vi "Begin.vi"(8 "error in":errorcluster) -> (0 "error out":errorcluster)   [LabVIEW 2016]
doc: "Called before other user functions, this VI is expected to open initial I/O refnums, load in file data, and do all program initialization. Notice that the <B>error out</B> terminal is simply used for data flow. Wiring it to other structures or subVIs ensures that this VI runs first."
uses:
  <vilib>/Rock Robotics/WPI/DriverStation/WPI_DriverStationRobotMode2.ctl
  <vilib>/Rock Robotics/WPI/Joystick/WPI_JoystickDeviceEnum.ctl
  <vilib>/Rock Robotics/SystemInterfaces/AI/FPGA_AIChannel.ctl
  <vilib>/Rock Robotics/SystemInterfaces/DIO/FPGA_DIOPWMChannel.ctl
  <vilib>/Rock Robotics/WPI/ThirdParty/CanMotor/TalonSRX/WPI_CANTalonSRX_APIControlMode.ctl
  <vilib>/Rock Robotics/WPI/ThirdParty/CanMotor/TalonSRX/WPI_CANTalonSRX_BrakeOverride.ctl
  <vilib>/Rock Robotics/SystemInterfaces/AI/FPGA_AIGyroChannel.ctl
  <vilib>/Rock Robotics/Network Tables/NT Write String Array.vi
  Robot Global Data.vi
  <vilib>/Rock Robotics/WPI/MotorControl/WPI_MotorControlOpen SPARK.vi
  <vilib>/Rock Robotics/Network Tables/NT Write Boolean.vi
  <vilib>/Rock Robotics/WPI/Ultrasonic/WPI_SonarMB1010AnalogOpen.vi
  <vilib>/Rock Robotics/WPI/Ultrasonic/WPI_SonarMB1010AnalogRefNum Registry Set.vi
  <vilib>/Rock Robotics/WPI/Switch/WPI_SwitchOpenLimit.vi
  <vilib>/Rock Robotics/SystemInterfaces/DIO/FPGA_DIOChannel.ctl
  2039lib.lvlib
panel:
  in  "Robot Mode":T1
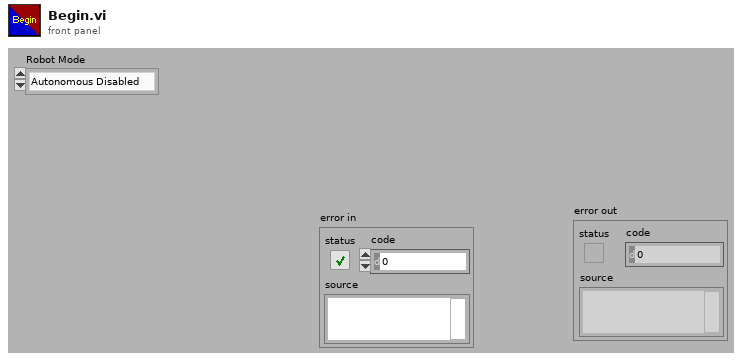
[diagram p1: front panel]
types:
  T1 = typedef "WPI_DriverStationRobotMode2.ctl" = enum16{"Autonomous Disabled", "Autonomous Enabled", "Teleop Disabled", "Teleop Enabled", "Disconnected", "Finish", "Test Disabled", "Test Enabled", "Emergency Stopped"}
  T2 = typedef "FPGA_DIOPWMChannel.ctl" = enum8{"PWM 0", "PWM 1", "PWM 2", "PWM 3", "PWM 4", "PWM 5", "PWM 6", "PWM 7", "PWM 8", "PWM 9", "PWM MXP 0", "PWM MXP 1", "PWM MXP 2", "PWM MXP 3", "PWM MXP 4", "PWM MXP 5", "PWM MXP 6", "PWM MXP 7", "PWM MXP 8", "PWM MXP 9", "Invalid"}
  T3 = enum16{"Driver Control", "Gear Coarse Adjust", "Gear Fine Adjust"}
  T4 = typedef "FPGA_AIGyroChannel.ctl" = enum8{"AI 0", "AI 1", "Invalid"}
  T5 = typedef "WPI_CANTalonSRX_BrakeOverride.ctl" = enum8{"No Override", "Override to Coast", "Override to Brake"}
  T6 = typedef "WPI_CANTalonSRX_APIControlMode.ctl" = enum8{"Percent VBus", "Speed", "Position", "Slave", "Unchanged / Invalid", "Voltage Compensation", "Current", "Motion Profile", "Motion Magic"}
  T7 = typedef "WPI_JoystickDeviceEnum.ctl" = enum16{"USB 0", "USB 1", "USB 2", "USB 3", "USB 4", "USB 5"}
  T8 = typedef "FPGA_AIChannel.ctl" = enum8{"AI 0", "AI 1", "AI 2", "AI 3", "AI MXP 0", "AI MXP 1", "AI MXP 2", "AI MXP 3", "Invalid"}
  T9 = typedef "WPI_MotorControlDeviceRef.ctl" = cluster{"DeviceStatus":errorcluster, "Type":T10, "PWM":cluster{"PWM Channel":T2, "DeadBand":T11}, "CAN":cluster{"Device Number":u8, "SetOutput VI Ref":variant, "GetOutput VI Ref":variant, "Enable VI Ref":variant, "Disable VI Ref":variant, "Data":variant}, "Invert":bool}
  T10 = typedef "WPI_MotorControlType.ctl" = enum16{"PWM", "CAN"}
  T11 = typedef "WPI_PWMDeadband.ctl" = cluster{"Name":string, "maxPositivePwm":i32, "minPositivePwm":i32, "centerPwm":i32, "maxNegativePwm":i32, "minNegativePwm":i32, "angularRange":u16}
  T12 = typedef "FPGA_DIOChannel.ctl" = enum8{"DIO 0", "DIO 1", "DIO 2", "DIO 3", "DIO 4", "DIO 5", "DIO 6", "DIO 7", "DIO 8", "DIO 9", "DIO MXP 0", "DIO MXP 1", "DIO MXP 2", "DIO MXP 3", "DIO MXP 4", "DIO MXP 5", "DIO MXP 6", "DIO MXP 7", "DIO MXP 8", "DIO MXP 9", "DIO MXP 10", "DIO MXP 11", "DIO MXP 12", "DIO MXP 13", "DIO MXP 14", "DIO MXP 15", "SPI Port CS1", "SPI Port CS2", "SPI Port CS3", "SPI Port MISO", "SPI Port MOSI", "Invalid"}
  T13 = typedef "WPI_DigitalInputDevRef.ctl" = cluster{"DevStatus":errorcluster, "DIO Channel":T12}
  T14 = typedef "WPI_SwitchDevRef.ctl" = cluster{"DevStatus":errorcluster, "DIO Channel":T12, "CntIndex":T15, "Normally Closed":bool}
  T15 = typedef "FPGA_CounterCtrSystemIndex.ctl" = enum8{"Ctr 0", "Ctr 1", "Ctr 2", "Ctr 3", "Ctr 4", "Ctr 5", "Ctr 6", "Ctr 7", "Invalid"}
  T16 = typedef "WPI_JoystickDevRef.ctl" = cluster{"Device":T7}
  T17 = typedef "WPI_SonarMB1010AnalogDeviceRef.ctl" = cluster{"AIDeviceRef":T18, "Scaling factor (V/in)":dbl, "Average Bits":u8}
  T18 = typedef "WPI_AnalogChannelDevRef.ctl" = cluster{"DevStatus":errorcluster, "Analog Channel":T8}
  T19 = typedef "WPI_ServoDeviceRef.ctl" = cluster{"DeviceStatus":errorcluster, "PWM Channel":T2, "DeadBand":T11}
  T20 = typedef "WPI_GyroDevRef.ctl" = cluster{"DevStatus":errorcluster, "Analog Channel":T8, "Offset":dbl, "Gain (VoltsPerDegree/Second)":dbl, "Gyro Type":enum16{"Analog", "XRS450"}, "Handle":i32, "SPI Bus":T21, "Device Found":bool, "Sample Rate":dbl, "Calibrate On Open":bool}
  T21 = typedef "spi_bus.ctl" = enum16{"SPI On-Board, CS0", "SPI On-Board, CS1", "SPI On-Board, CS2", "SPI On-Board, CS3", "SPI MXP", "Invalid"}
  T22 = typedef "WPI_AccelerometerDevRef.ctl" = cluster{"DevStatus":errorcluster, "Scaling":T23, "Analog Channels":T24, "I2C Bus":T25, "SPI Bus":T21, "Accel Range":T26, "ADXL Axes":T27, "Handle":i32, "Device Address":u8, "Accel Type":enum16{"Analog", "ADXL345 I2C", "ADXL345 SPI", "Internal", "ADXL362 SPI"}}
  T23 = typedef "WPI_AccelerometerScaling.ctl" = cluster{"Gain (VoltsPerG)":dbl, "Center Voltage":dbl}
  T24 = typedef "WPI_AccelerometerAnalogChannels.ctl" = cluster{"X-Axis":T8, "Y-Axis":T8, "Z-Axis":T8}
  T25 = typedef "i2c_bus.ctl" = enum16{"I2C On-Board", "I2C MXP", "Invalid"}
  T26 = typedef "ADXL345 Range.ctl" = u8
  T27 = typedef "WPI_AccelerometerADXL345 Axes.ctl" = cluster{"X-Axis":bool, "Y-Axis":bool, "Z-Axis":bool}
  T28 = cluster{"GyroDevRef":T20, "AccelerometerDevRef":T22}
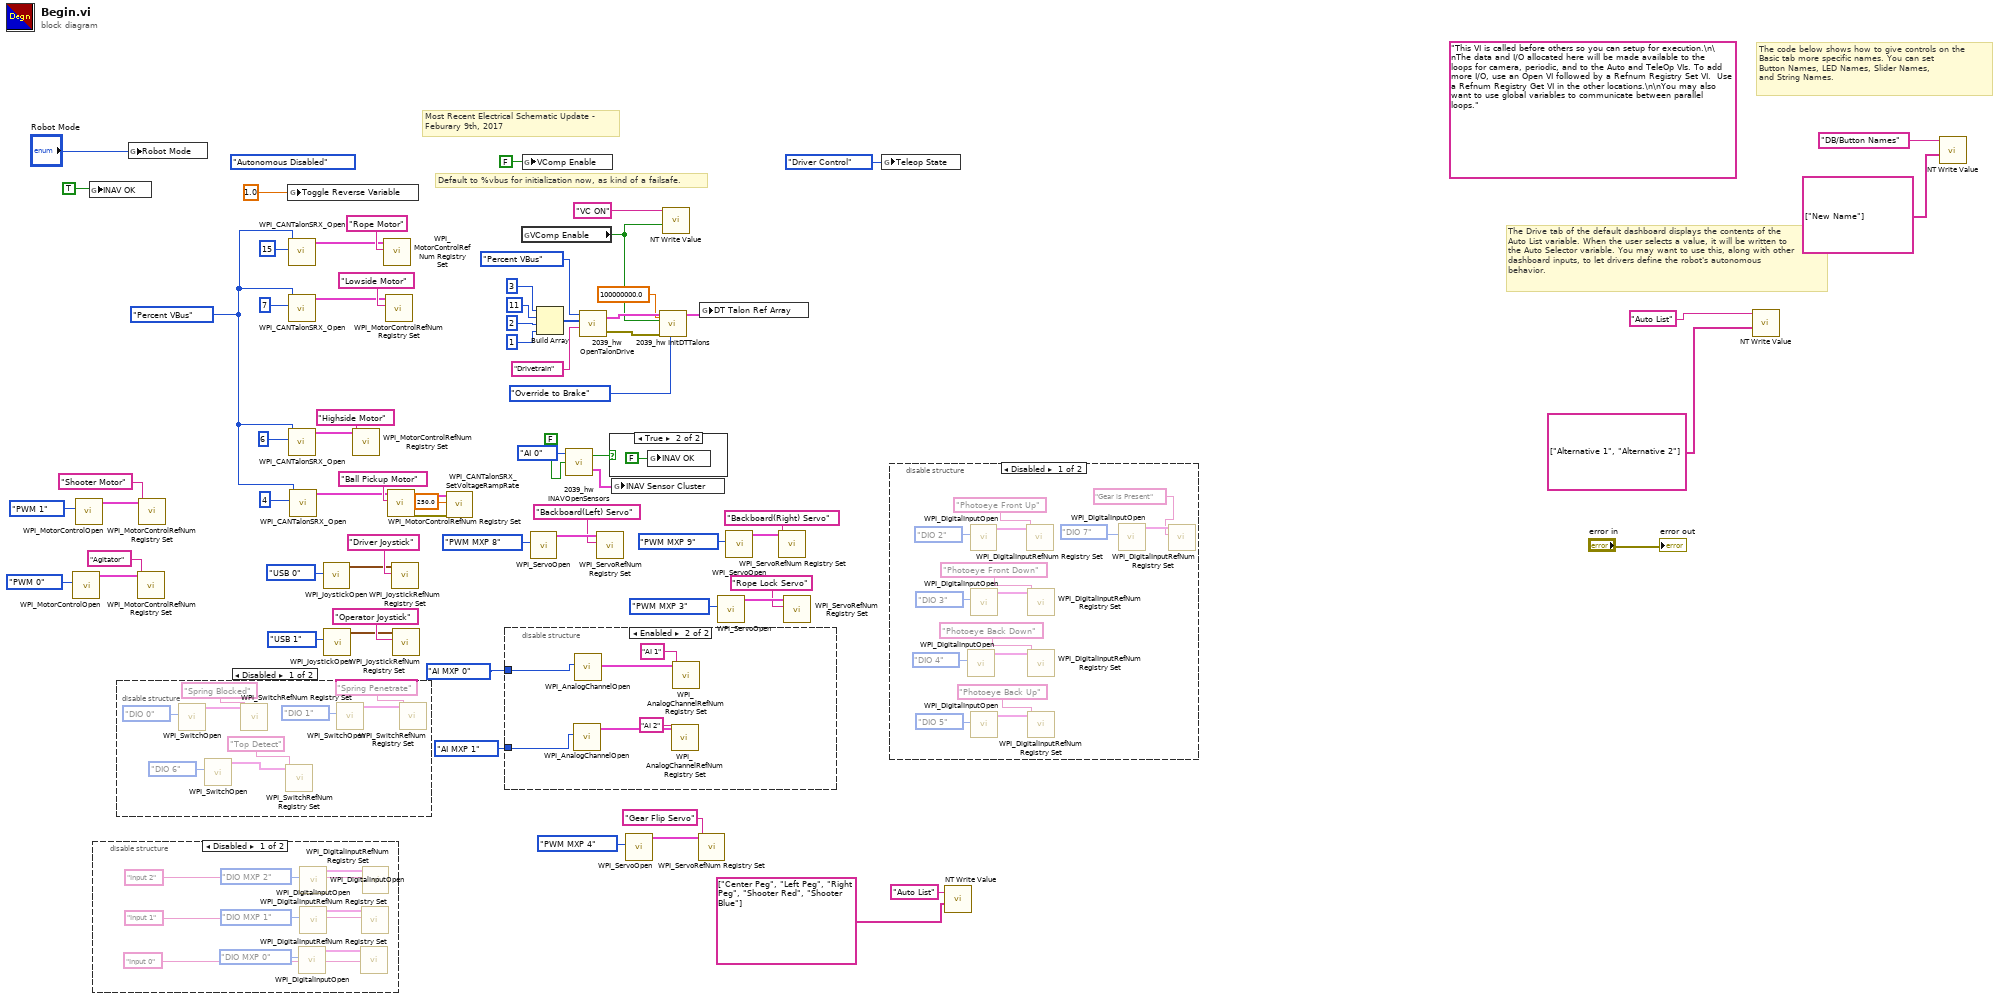
[diagram p0: block diagram]
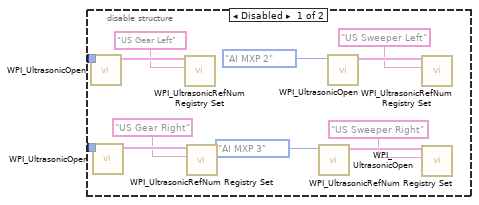
[diagram p4: hidden frame]
diagram:
  w50 = WPI_CANTalonSRX_APIControlMode."Percent VBus" ("Control Mode")
  (unwired) WPI_DriverStationRobotMode2."Autonomous Disabled" ("Robot Mode")
  (unwired) "This VI is called before others so you can setup for execution.\n\nThe data and I/O allocated here will be made available to the loops for camera, periodic, and to the Auto and TeleOp VIs. To add more I/O, use an Open VI followed by a Refnum Registry Set VI.  Use a Refnum Registry Get VI in the other locations.\n\nYou may also want to use global variables to communicate between parallel loops."
  # "Default to %vbus for initialization now, as kind of a failsafe."
  # "Most Recent Electrical Schematic Update -\nFeburary 9th, 2017"
  # "The Drive tab of the default dashboard displays the contents of the\nAuto List variable. When the user selects a value, it will be written to\nthe Auto Selector variable. You may want to use this, along with other\ndashboard inputs, to let drivers define the robot's autonomous\nbehavior."
  # "The code below shows how to give controls on the\nBasic tab more specific names. You can set\nButton Names, LED Names, Slider Names,\nand String Names."
  n1 = call-poly <vilib>:"WPI_MotorControlOpen.vi"("PWM Channel"=FPGA_DIOPWMChannel."PWM 0") -> ("MotorControlDeviceRef"=w6:T9)  [unwired: 9 in, 1 out]
  n2 = call-poly <vilib>:"WPI_MotorControlOpen.vi"("PWM Channel"=FPGA_DIOPWMChannel."PWM 1") -> ("MotorControlDeviceRef"=w7:T9)  [unwired: 9 in, 1 out]
  n3 = global write "Robot Global Data.vi" "INAV OK"(TRUE) -> ()
  n4 = disable-structure shown="Disabled" {
    frame Disabled {
      n5 = call <vilib>:"WPI_DigitalInputOpen.vi"("DIO Channel"=FPGA_DIOChannel."DIO MXP 0") -> ("DigitalInputDevRef"=w77:T13)  [unwired: 9 in, 1 out]
      n6 = call <vilib>:"WPI_DigitalInputOpen.vi"("DIO Channel"=FPGA_DIOChannel."DIO MXP 2") -> ("DigitalInputDevRef"=w76:T13)  [unwired: 9 in, 1 out]
      n7 = call <vilib>:"WPI_DigitalInputOpen.vi"("DIO Channel"=FPGA_DIOChannel."DIO MXP 1") -> ("DigitalInputDevRef"=w78:T13)  [unwired: 9 in, 1 out]
      n8 = call <vilib>:"WPI_DigitalInputRefNum Registry Set.vi"("refnum name"="Input 0", "DigitalInputDevRef"=w77) -> ()  [unwired: 8 in, 2 out]
      n9 = call <vilib>:"WPI_DigitalInputRefNum Registry Set.vi"("refnum name"="Input 1", "DigitalInputDevRef"=w78) -> ()  [unwired: 8 in, 2 out]
      n10 = call <vilib>:"WPI_DigitalInputRefNum Registry Set.vi"("refnum name"="Input 2", "DigitalInputDevRef"=w76) -> ()  [unwired: 8 in, 2 out]
    }
    frame Enabled {
    }
  }
  n11 = disable-structure shown="Disabled" {
    frame Disabled {
      n12 = call-poly <vilib>:"WPI_SwitchOpen.vi"("DIO Channel"=FPGA_DIOChannel."DIO 0") -> ("SwitchDevRef"=w90:T14)  [unwired: 9 in, 1 out]
      n13 = call-poly <vilib>:"WPI_SwitchOpen.vi"("DIO Channel"=FPGA_DIOChannel."DIO 6") -> ("SwitchDevRef"=w84:T14)  [unwired: 9 in, 1 out]
      n14 = call <vilib>:"WPI_SwitchRefNum Registry Set.vi"("refnum name"="Spring Blocked", "SwitchDevRef"=w90) -> ()  [unwired: 8 in, 2 out]
      n15 = call <vilib>:"WPI_SwitchRefNum Registry Set.vi"("refnum name"="Top Detect", "SwitchDevRef"=w84) -> ()  [unwired: 8 in, 2 out]
      n16 = call-poly <vilib>:"WPI_SwitchOpen.vi"("DIO Channel"=FPGA_DIOChannel."DIO 1") -> ("SwitchDevRef"=w87:T14)  [unwired: 9 in, 1 out]
      n17 = call <vilib>:"WPI_SwitchRefNum Registry Set.vi"("refnum name"="Spring Penetrate", "SwitchDevRef"=w87) -> ()  [unwired: 8 in, 2 out]
    }
    frame Enabled {
    }
  }
  n18 = global write "Robot Global Data.vi" "Robot Mode"("Robot Mode") -> ()
  n19 = call <vilib>:"WPI_MotorControlRefNum Registry Set.vi"("refnum name"="Agitator", "MotorControlDevRef"=w6) -> ()  [unwired: 8 in, 2 out]
  n20 = call <vilib>:"WPI_MotorControlRefNum Registry Set.vi"("refnum name"="Shooter Motor", "MotorControlDevRef"=w7) -> ()  [unwired: 8 in, 2 out]
  n21 = global write "Robot Global Data.vi" "Toggle Reverse Variable"(1.0 ("Toggle Reverse Variable")) -> ()
  n22 = call <vilib>:"WPI_CANTalonSRX_Open.vi"("Device Number"=15, "Control Mode"=w50) -> ("CAN Talon SRX Ref"=w44:T9)  [unwired: 8 in, 1 out]
  n23 = call <vilib>:"WPI_CANTalonSRX_Open.vi"("Device Number"=7, "Control Mode"=w50) -> ("CAN Talon SRX Ref"=w43:T9)  [unwired: 8 in, 1 out]
  n24 = call <vilib>:"WPI_CANTalonSRX_Open.vi"("Device Number"=6, "Control Mode"=w50) -> ("CAN Talon SRX Ref"=w42:T9)  [unwired: 8 in, 1 out]
  n25 = call <vilib>:"WPI_CANTalonSRX_Open.vi"("Device Number"=4, "Control Mode"=w50) -> ("CAN Talon SRX Ref"=w41:T9)  [unwired: 8 in, 1 out]
  n26 = call <vilib>:"WPI_JoystickOpen.vi"("JoystickDevice"=WPI_JoystickDeviceEnum."USB 0") -> ("JoystickDevRef"=w71:T16)  [unwired: 10 in]
  n27 = call <vilib>:"WPI_JoystickOpen.vi"("JoystickDevice"=WPI_JoystickDeviceEnum."USB 1") -> ("JoystickDevRef"=w61:T16)  [unwired: 10 in]
  n28 = call <vilib>:"WPI_MotorControlRefNum Registry Set.vi"("refnum name"="Highside Motor", "MotorControlDevRef"=w42) -> ()  [unwired: 8 in, 2 out]
  n29 = call <vilib>:"WPI_MotorControlRefNum Registry Set.vi"("refnum name"="Rope Motor", "MotorControlDevRef"=w44) -> ()  [unwired: 8 in, 2 out]
  n30 = call <vilib>:"WPI_MotorControlRefNum Registry Set.vi"("refnum name"="Lowside Motor", "MotorControlDevRef"=w43) -> ()  [unwired: 8 in, 2 out]
  n31 = call <vilib>:"WPI_MotorControlRefNum Registry Set.vi"("refnum name"="Ball Pickup Motor", "MotorControlDevRef"=w41) -> ("error out"=w11:errorcluster, "MotorControlDevRef"=w12:T9)  [unwired: 8 in]
  n32 = call <vilib>:"WPI_JoystickRefNum Registry Set.vi"("refnum name"="Driver Joystick", "JoystickDevRef"=w71) -> ()  [unwired: 8 in, 2 out]
  n33 = call <vilib>:"WPI_JoystickRefNum Registry Set.vi"("refnum name"="Operator Joystick", "JoystickDevRef"=w61) -> ()  [unwired: 8 in, 2 out]
  n34 = call <vilib>:"WPI_CANTalonSRX_SetVoltageRampRate.vi"("error in (no error)"=w11, "Throttle Ramp Rate (percent/s)"=250.0, "CAN Talon SRX Ref"=w12) -> ()  [unwired: 7 in, 2 out]
  n35 = disable-structure shown="Enabled" {
    disable-tunnel: FPGA_AIChannel."AI MXP 0" ("Analog Channel") -> [w102 w107]
    disable-tunnel: FPGA_AIChannel."AI MXP 1" ("Analog Channel") -> [w99 w108]
    frame Disabled {
      n36 = call-poly <vilib>:"WPI_UltrasonicOpen.vi"("Analog Channel"=w102) -> ("SonarMB1010AnalogDevRef"=w101:T17)  [unwired: 9 in, 1 out]
      n37 = call-poly <vilib>:"WPI_UltrasonicOpen.vi"("Analog Channel"=w99) -> ("SonarMB1010AnalogDevRef"=w98:T17)  [unwired: 9 in, 1 out]
      n38 = call-poly <vilib>:"WPI_UltrasonicRefNum Registry Set.vi"("refnum name"="US Gear Left", "SonarMB1010AnalogDevRef"=w101) -> ()  [unwired: 8 in, 2 out]
      n39 = call-poly <vilib>:"WPI_UltrasonicRefNum Registry Set.vi"("refnum name"="US Gear Right", "SonarMB1010AnalogDevRef"=w98) -> ()  [unwired: 8 in, 2 out]
      n40 = call-poly <vilib>:"WPI_UltrasonicOpen.vi"("Analog Channel"=FPGA_AIChannel."AI MXP 3") -> ("SonarMB1010AnalogDevRef"=w92:T17)  [unwired: 9 in, 1 out]
      n41 = call-poly <vilib>:"WPI_UltrasonicOpen.vi"("Analog Channel"=FPGA_AIChannel."AI MXP 2") -> ("SonarMB1010AnalogDevRef"=w95:T17)  [unwired: 9 in, 1 out]
      n42 = call-poly <vilib>:"WPI_UltrasonicRefNum Registry Set.vi"("refnum name"="US Sweeper Left", "SonarMB1010AnalogDevRef"=w95) -> ()  [unwired: 8 in, 2 out]
      n43 = call-poly <vilib>:"WPI_UltrasonicRefNum Registry Set.vi"("refnum name"="US Sweeper Right", "SonarMB1010AnalogDevRef"=w92) -> ()  [unwired: 8 in, 2 out]
    }
    frame Enabled {
      n44 = call <vilib>:"WPI_AnalogChannelOpen.vi"("Analog Channel"=w108) -> ("AIDeviceRef"=w106:T18)  [unwired: 9 in, 1 out]
      n45 = call <vilib>:"WPI_AnalogChannelOpen.vi"("Analog Channel"=w107) -> ("AIDeviceRef"=w105:T18)  [unwired: 9 in, 1 out]
      n46 = call <vilib>:"WPI_AnalogChannelRefNum Registry Set.vi"("refnum name"="AI 2", "AIDeviceRef"=w106) -> ()  [unwired: 8 in, 2 out]
      n47 = call <vilib>:"WPI_AnalogChannelRefNum Registry Set.vi"("refnum name"="AI 1", "AIDeviceRef"=w105) -> ()  [unwired: 8 in, 2 out]
    }
  }
  n48 = global read "Robot Global Data.vi" "VComp Enable"() -> (w17:bool)
  n49 = global write "Robot Global Data.vi" "VComp Enable"(FALSE) -> ()
  n50 = call <vilib>:"WPI_ServoOpen.vi"("PWM Channel"=FPGA_DIOPWMChannel."PWM MXP 8") -> ("ServoDeviceRef"=w20:T19)  [unwired: 9 in, 1 out]
  n51 = Build Array(u8 3 ("Device Number"), u8 11 ("Device Number"), u8 2 ("Device Number"), u8 1 ("Device Number")) -> (w34:u8[])
  n52 = call "2039_hw INAVOpenSensors.vi"("Use External Accel"=FALSE, "Gyroscope Analog Channel"=FPGA_AIGyroChannel."AI 0") -> ("INAV Sensor Cluster"=w1:T28, "INAV Not OK"=w24:bool)  [unwired: 1 in]
  n53 = call "2039_hw OpenTalonDrive.vi"("refnum name"="Drivetrain", "CAN IDs"=w34, "Control Mode"=WPI_CANTalonSRX_APIControlMode."Percent VBus") -> ("error out"=w30:errorcluster, "Drivetrain Talon SRX Ref Array"=w31:T9[])  [unwired: 1 in]
  n54 = call <vilib>:"WPI_ServoRefNum Registry Set.vi"("refnum name"="Backboard(Left) Servo", "ServoDeviceRef"=w20) -> ()  [unwired: 8 in, 2 out]
  n55 = case shown="True" w24 {
    frame False {
    }
    frame True {
      n56 = global write "Robot Global Data.vi" "INAV OK"(FALSE) -> ()
    }
  }
  n57 = global write "Robot Global Data.vi" "INAV Sensor Cluster"(w1) -> ()
  n58 = call <vilib>:"WPI_ServoOpen.vi"("PWM Channel"=FPGA_DIOPWMChannel."PWM MXP 4") -> ("ServoDeviceRef"=w14:T19)  [unwired: 9 in, 1 out]
  n59 = call "2039_hw InitDTTalons.vi"("Brake / Coast Mode"=WPI_CANTalonSRX_BrakeOverride."Override to Brake", "Ramp Rate (Percent/s)"=100000000.0, "error in (no error)"=w30, "Enable VComp"=w17, "DT Talon Ref Array"=w31) -> ("DT Talon Ref Array"=w22:T9[])  [unwired: 5 in, 1 out]
  n60 = call-poly <vilib>:"NT Write Value.vi"("Boolean"=w17, "Name"="VC ON") -> ()  [unwired: 9 in, 1 out]
  n61 = call <vilib>:"WPI_ServoRefNum Registry Set.vi"("refnum name"="Gear Flip Servo", "ServoDeviceRef"=w14) -> ()  [unwired: 8 in, 2 out]
  n62 = global write "Robot Global Data.vi" "DT Talon Ref Array"(w22) -> ()
  n63 = call <vilib>:"WPI_ServoOpen.vi"("PWM Channel"=FPGA_DIOPWMChannel."PWM MXP 3") -> ("ServoDeviceRef"=w55:T19)  [unwired: 9 in, 1 out]
  n64 = call <vilib>:"WPI_ServoOpen.vi"("PWM Channel"=FPGA_DIOPWMChannel."PWM MXP 9") -> ("ServoDeviceRef"=w21:T19)  [unwired: 9 in, 1 out]
  n65 = call <vilib>:"WPI_ServoRefNum Registry Set.vi"("refnum name"="Backboard(Right) Servo", "ServoDeviceRef"=w21) -> ()  [unwired: 8 in, 2 out]
  n66 = call <vilib>:"WPI_ServoRefNum Registry Set.vi"("refnum name"="Rope Lock Servo", "ServoDeviceRef"=w55) -> ()  [unwired: 8 in, 2 out]
  n67 = global write "Robot Global Data.vi" "Teleop State"(T3."Driver Control" ("Teleop State")) -> ()
  n68 = disable-structure shown="Disabled" {
    frame Disabled {
      n69 = call <vilib>:"WPI_DigitalInputOpen.vi"("DIO Channel"=FPGA_DIOChannel."DIO 4") -> ("DigitalInputDevRef"=w113:T13)  [unwired: 9 in, 1 out]
      n70 = call <vilib>:"WPI_DigitalInputOpen.vi"("DIO Channel"=FPGA_DIOChannel."DIO 2") -> ("DigitalInputDevRef"=w123:T13)  [unwired: 9 in, 1 out]
      n71 = call <vilib>:"WPI_DigitalInputOpen.vi"("DIO Channel"=FPGA_DIOChannel."DIO 3") -> ("DigitalInputDevRef"=w120:T13)  [unwired: 9 in, 1 out]
      n72 = call <vilib>:"WPI_DigitalInputOpen.vi"("DIO Channel"=FPGA_DIOChannel."DIO 5") -> ("DigitalInputDevRef"=w115:T13)  [unwired: 9 in, 1 out]
      n73 = call <vilib>:"WPI_DigitalInputRefNum Registry Set.vi"("refnum name"="Photoeye Front Up", "DigitalInputDevRef"=w123) -> ()  [unwired: 8 in, 2 out]
      n74 = call <vilib>:"WPI_DigitalInputRefNum Registry Set.vi"("refnum name"="Photoeye Front Down", "DigitalInputDevRef"=w120) -> ()  [unwired: 8 in, 2 out]
      n75 = call <vilib>:"WPI_DigitalInputRefNum Registry Set.vi"("refnum name"="Photoeye Back Down", "DigitalInputDevRef"=w113) -> ()  [unwired: 8 in, 2 out]
      n76 = call <vilib>:"WPI_DigitalInputRefNum Registry Set.vi"("refnum name"="Photoeye Back Up", "DigitalInputDevRef"=w115) -> ()  [unwired: 8 in, 2 out]
      n77 = call <vilib>:"WPI_DigitalInputOpen.vi"("DIO Channel"=FPGA_DIOChannel."DIO 7") -> ("DigitalInputDevRef"=w111:T13)  [unwired: 9 in, 1 out]
      n78 = call <vilib>:"WPI_DigitalInputRefNum Registry Set.vi"("refnum name"="Gear is Present", "DigitalInputDevRef"=w111) -> ()  [unwired: 8 in, 2 out]
    }
    frame Enabled {
    }
  }
  n79 = call-poly <vilib>:"NT Write Value.vi"("String Array"=string[] ["Center Peg", "Left Peg", "Right Peg", "Shooter Red", "Shooter Blue"], "Name"="Auto List") -> ()  [unwired: 9 in, 1 out]
  n80 = call-poly <vilib>:"NT Write Value.vi"("String Array"=string[] ["Alternative 1", "Alternative 2"], "Name"="Auto List") -> ()  [unwired: 9 in, 1 out]
  n81 = call-poly <vilib>:"NT Write Value.vi"("String Array"=string[] ["New Name"], "Name"="DB/Button Names") -> ()  [unwired: 9 in, 1 out]
  "error out" <- "error in"
